vi "Log Action.vi"(4 "Log Map in":refnum<class "LogMap.lvclass">, 8 "error in (no error)":errorcluster, 9 "object in":refnum<class>, 10 "ActionType":string, 11 "SqlMapper in":refnum<class "SqlMapper.lvclass">) -> (0 "error out":errorcluster, 3 "SqlMapper out":refnum<class "SqlMapper.lvclass">)   [LabVIEW 2024, in "ORM.lvlib" / "LogMap.lvclass"]
uses:
  LogMap.lvclass
  C:/Viviota/Projects/R&D/__OpenSource/VIV_ORM/ORM/TypeMap/TypeMap.lvclass
  ORM/SqlMapper/SqlMapper.lvclass
  LogMap.lvclass/LogMap.ctl
  ORM/TypeMap/TypeMap.lvclass
  ORM/TypeMap/TypeMap.lvclass/TypeMap.ctl
  ORM/TypeMap/Read Autokey.vi
  Read IncludeObjRepresentation.vi
  ORM/TypeMap/Write ExplicitFieldOrder.vi
  ORM/TypeMap/Read Table Name.vi
  ORM/TypeMap/Write Table Name.vi
  <vilib>/JDP Science/JSONtext/JSONtext.lvlib
  <vilib>/Viviota/shared/ORM_lib.lvlibp/ObjectRow/ObjectLUT.lvclass
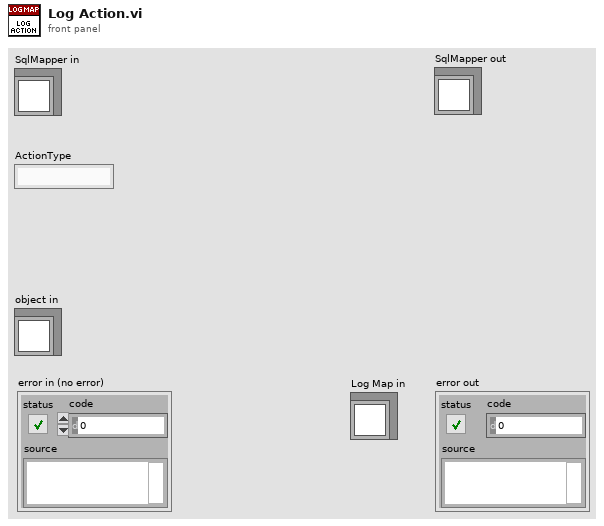
[diagram p1: front panel]
types:
  T1 = typedef "ORM.lvlib/LogMap.lvclass/logmapcluster.ctl" = cluster{"ActionTime":timestamp, "ActionType":string, "ObjectTable":string, "ObjectId":i64, "ObjectRepr":string, "Username":string, "Domain":string, "IP":string, "MachineGuid":string}
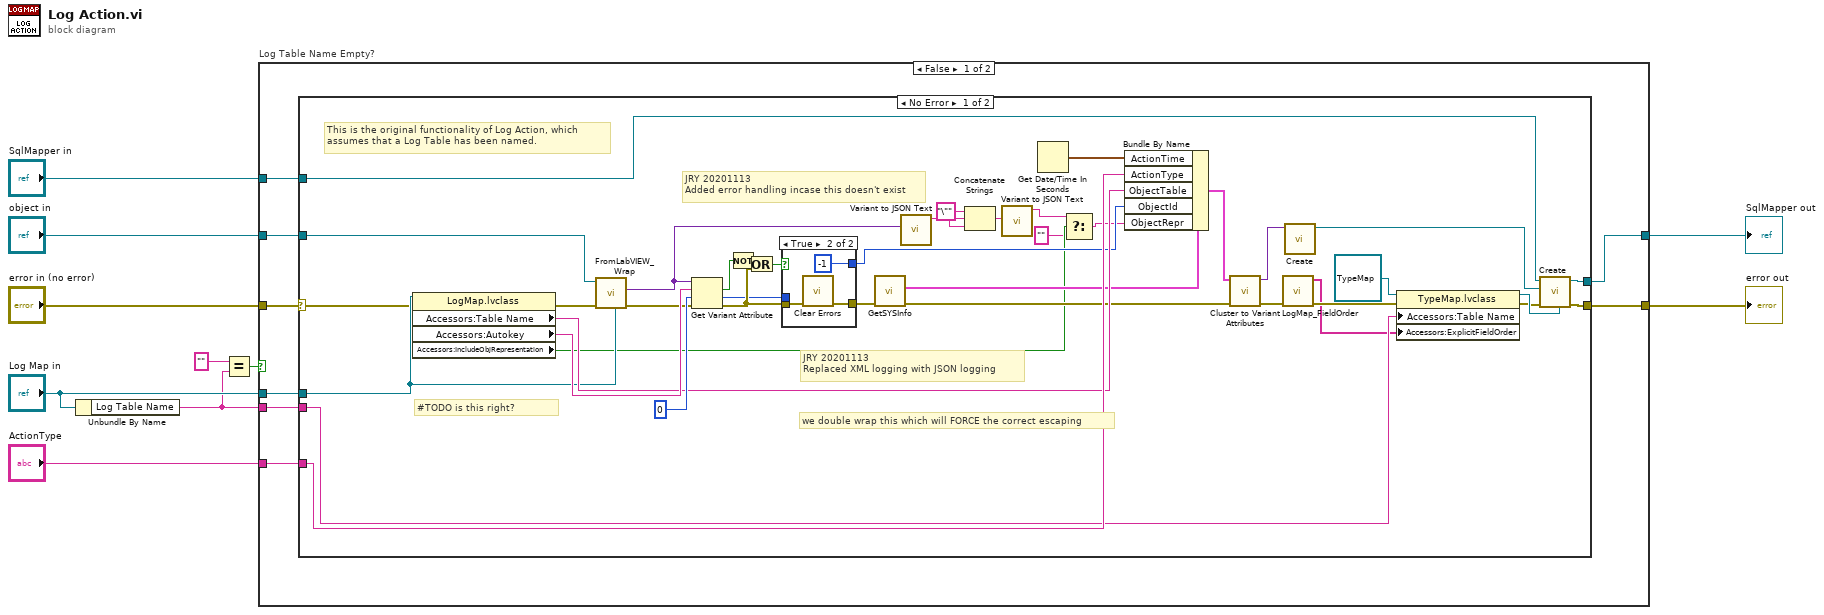
[diagram p0: block diagram]
diagram:
  n1 = Unbundle By Name("Log Map in") -> ("Log Table Name"=w1:string)
  n2 = Equal?(x="", y=w1) -> (x = y?=w2:bool)
  n3 = case "Log Table Name Empty?" shown="False" w2 {
    tunnel: "ActionType" -> [w18 _]
    tunnel: "object in" -> [w17 _]
    tunnel: [w16 w67] -> w8
    tunnel: "SqlMapper in" -> [w15 w67]
    tunnel: [w14 w66] -> w6
    tunnel: "error in (no error)" -> [w13 w66]
    tunnel: "Log Map in" -> [w12 _]
    tunnel: w1 -> [w11 _]
    frame False {
      n4 = case shown="No Error" w13 {
        selector: w13 -> [w34 w65]
        tunnel: w12 -> [w49 _]
        tunnel: w17 -> [w50 _]
        tunnel: w15 -> [w25 w64]
        tunnel: [w58 w65] -> w14
        tunnel: [w57 w64] -> w16
        tunnel: w18 -> [w54 _]
        tunnel: w11 -> [w43 _]
        frame No Error {
          w31 = "\"" ("string")
          # "we double wrap this which will FORCE the correct escaping"
          # "JRY 20201113\nAdded error handling incase this doesn't exist"
          # "JRY 20201113 \nReplaced XML logging with JSON logging"
          # "This is the original functionality of Log Action, which \nassumes that a Log Table has been named."
          # "#TODO is this right?"
          n5 = property class="LogMap.lvclass"(reference=w49, error in=w34) -> (error out=w47:errorcluster, "Accessors:Table Name"=w51:string, "Accessors:Autokey"=w53:string, "Accessors:IncludeObjRepresentation"=w20:bool)  [unwired: 1 out]
          n6 = call "FromLabVIEW_Wrap.vi"("TypeMap in"=w49, "error in (no error)"=w47, "object in"=w50) -> ("error out"=w48:errorcluster, "DbRow"=w42:variant)  [unwired: 7 in]
          n7 = Get Variant Attribute(Variant=w42, name=w53, default value (empty Variant)=i64 0 ("ObjectId"), error in=w48) -> (found=w41:bool, value=w36:i64, error out=w38:errorcluster)  [unwired: 1 out]
          n8 = Not(x=w41) -> (.not. x?=w40:bool)
          n9 = Or(x=w40, y=w38) -> (x .or. y?=w39:bool)
          n10 = case shown="True" w39 {
            tunnel: w38 -> [w59 w62]
            tunnel: [w60 -1] -> w37
            tunnel: w36 -> [w60 _]
            tunnel: [w59 w61] -> w35
            frame False {
            }
            frame True {
              n11 = call <vilib>:"Clear Errors.vi"("error in (no error)"=w62) -> ("error out"=w61:errorcluster)  [unwired: 5 in, 1 out]
            }
          }
          n12 = call "GetSYSInfo.vi"("error in (no error)"=w35) -> ("error out"=w46:errorcluster, "Info"=w30:T1)  [unwired: 9 in]
          n13 = call <vilib>:"Variant to JSON Text.vi"("Variant"=w42) -> ("<JSON>"=w32:string)  [unwired: 8 in, 2 out]
          n14 = Concatenate Strings(w31, w32, w31) -> (w29:string)
          n15 = call <vilib>:"Variant to JSON Text.vi"("Variant"=w29) -> ("<JSON>"=w21:string)  [unwired: 8 in, 2 out]
          n16 = Get Date/Time In Seconds() -> (seconds since 1Jan1904=w33:timestamp)
          n17 = Select(t=w21, s=w20, f="") -> (s? t:f=w22:string)
          n18 = Bundle By Name(cluster=w30, "ActionTime"=w33, "ActionType"=w54, "ObjectTable"=w51, "ObjectId"=w37, "ObjectRepr"=w22) -> (w44:T1)
          n19 = call "Cluster to Variant Attributes.vi"("error in (no error)"=w46, "Cluster"=w44) -> ("error out"=w28:errorcluster, "Variant"=w24:variant)  [unwired: 8 in]
          n20 = call "LogMap_FieldOrder.vi"("Error In"=w28) -> ("Error Out"=w27:errorcluster, "FieldOrder out"=w26:string[])  [unwired: 9 in]
          n21 = call <vilib>:"Create.vi"("LUT"=w24) -> ("ORM_lib.lvlib:ObjectLUT.lvclass"=w23:refnum<class "ObjectLUT.lvclass">)  [unwired: 9 in, 1 out]
          n22 = property class="TypeMap.lvclass"(reference=refnum<class "TypeMap.lvclass"> refnum ("TypeMap in"), error in=w27, "Accessors:Table Name"=w43, "Accessors:ExplicitFieldOrder"=w26) -> (reference out=w55:refnum<class "TypeMap.lvclass">, error out=w45:errorcluster)
          n23 = call-dynamic <vilib>:"Create.vi"("TypeMap in"=w55, "error in (no error)"=w45, "object in"=w23, "SqlMapper in"=w25) -> ("error out"=w58:errorcluster, "SqlMapper out"=w57:refnum<class "SqlMapper.lvclass">)  [unwired: 4 in, 2 out]
        }
        frame Error {
        }
      }
    }
    frame True {
      # "When the Log Table name is an empty string, \nthen no logging action will occur."
    }
  }
  "SqlMapper out" <- w8
  "error out" <- w6
